vi "Dashboard_Serial.vi"() -> ()   [LabVIEW 2025]
uses:
  <vilib>/Instr/_visa.llb/VISA Open Access Mode.ctl
  Cluster.ctl
  <vilib>/Instr/_visa.llb/VISA Configure Serial Port (Instr).vi
panel:
  out "return count":u32
  out "error out":errorcluster
  out "value":T1
  in  "stop":bool
  in  "VISA resource name":refnum<visa-resource-name>
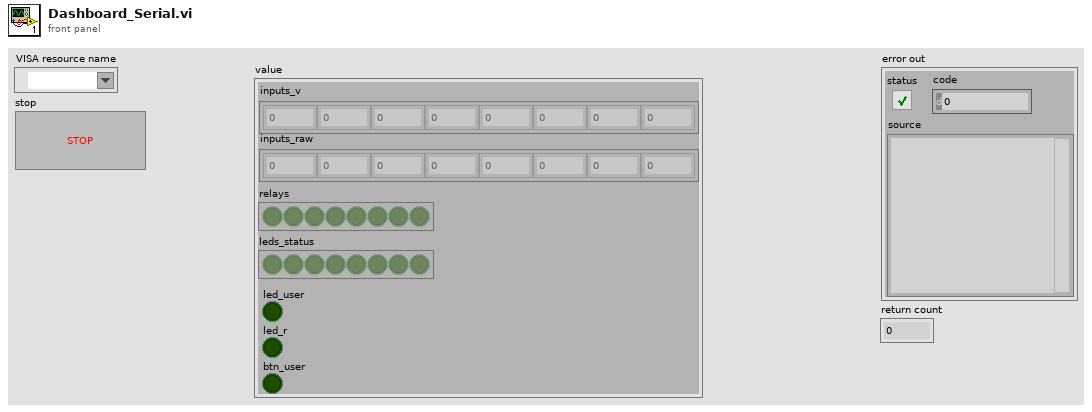
[diagram p1: front panel]
types:
  T1 = cluster{"relays":bool[], "leds_status":bool[], "led_user":bool, "led_r":bool, "btn_user":bool, "inputs_v":dbl[], "inputs_raw":i32[]}
  T2 = typedef "VISA Open Access Mode.ctl" = u32
  T3 = typedef "Cluster.ctl" = cluster{"relays":bool[], "leds_status":bool[], "led_user":bool, "led_r":bool, "btn_user":bool, "inputs_v":dbl[], "inputs_raw":i32[]}
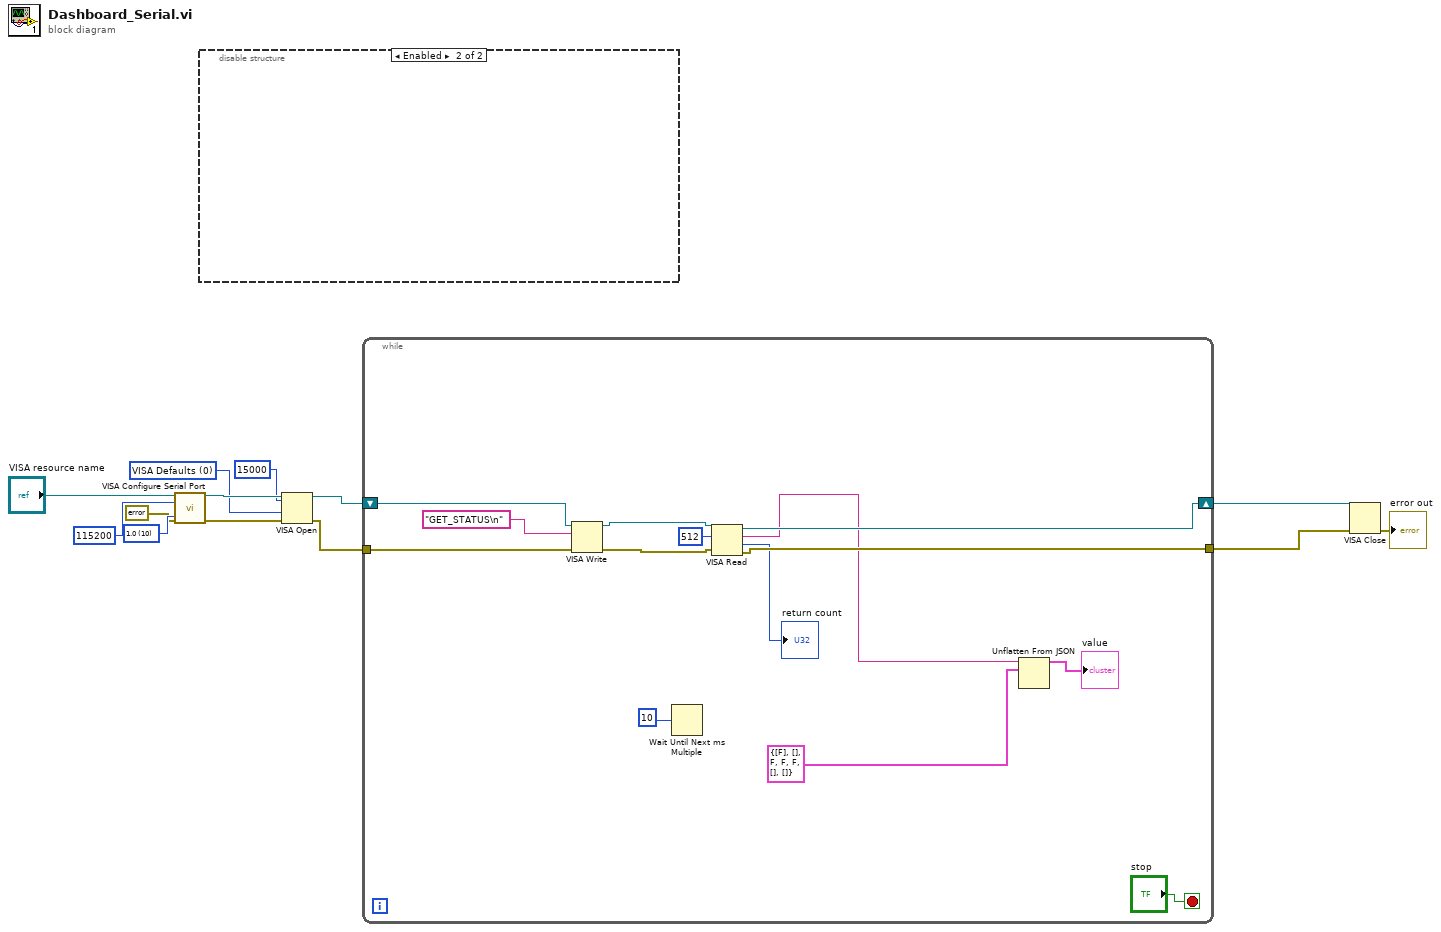
[diagram p0: block diagram]
diagram:
  w3 = T2 0 items=["VISA Defaults"=0, "Exclusive Lock"=1, "Load Configured Settings"=4] ("Access Mode")
  w5 = u16 10 items=["1.0"=10, "1.5"=15, "2.0"=20] ("stop bits (10: 1 bit)")
  n1 = call-poly "VISA Configure Serial Port"("VISA resource name"="VISA resource name", "baud rate (9600)"=u32 115200, "error in (no error)"=errorcluster {"status"=FALSE, "code"=0, "source"=""}, "stop bits (10: 1 bit)"=w5) -> ("VISA resource name out"=w8:refnum<visa-resource-name>, "error out"=w9:errorcluster)  [unwired: 10 in]
  n2 = disable-structure shown="Enabled" {
    frame Disabled {
    }
    frame Enabled {
    }
  }
  n3 = VISA Open(timeout (0)=u32 15000 ("VISA Open timeout (0)"), access mode=w3, error in (no error)=w9, VISA resource name=w8) -> (VISA resource name=w13:refnum<visa-resource-name>, error out=w11:errorcluster)  [unwired: 1 in]
  n4 = while {
    tunnel: [w24] -> w12
    tunnel: w11 -> [w22]
    shift-right: [w19] -> w1
    shift-left: w13 -> [w27]
    stop <- "stop" stop-if-true
    n5 = VISA Write(VISA resource name=w27, write buffer="GET_STATUS\n", error in (no error)=w22) -> (VISA resource name out=w26:refnum<visa-resource-name>, error out=w23:errorcluster)  [unwired: 1 out]
    n6 = Wait Until Next ms Multiple(millisecond multiple=u32 10 ("milliseconds to wait")) -> ()  [unwired: 1 out]
    n7 = VISA Read(VISA resource name=w26, byte count=u32 512, error in (no error)=w23) -> (VISA resource name out=w19:refnum<visa-resource-name>, read buffer=w17:string, return count=→"return count":u32, error out=w24:errorcluster)
    n8 = Unflatten From JSON(JSON string=w17, type and defaults=T3 {"relays"=[FALSE], "leds_status"=[], "led_user"=FALSE, "led_r"=FALSE, "btn_user"=FALSE, "inputs_v"=[], "inputs_raw"=[]} ("value 2")) -> (value=→"value":T3)  [unwired: 5 in, 1 out]
  }
  n9 = VISA Close(VISA resource name=w1, error in (no error)=w12) -> (error out=→"error out":errorcluster)
